vi "Auto Half Ratchet.vi"(9 "ServoDeviceRef":T11, 10 "ServoDeviceRef 2":T11, 11 "RobotDriveDevRef":T1) -> ()   [LabVIEW 2014]
uses:
  <vilib>/Rock Robotics/WPI/PWM/Servo/WPI_ServoDeviceRef.ctl
  <vilib>/Rock Robotics/SystemInterfaces/Typedef/FPGA_TypedefDigitalModule.ctl
  <vilib>/Rock Robotics/SystemInterfaces/DIO/FPGA_DIOPWMChannel.ctl
  <vilib>/Rock Robotics/WPI/PWM/WPI_PWMDeadband.ctl
  <vilib>/Rock Robotics/WPI/RobotDrive/WPI_RobotDriveDevRef.ctl
  <vilib>/Rock Robotics/WPI/MotorControl/WPI_MotorControlDeviceRef.ctl
  <vilib>/Rock Robotics/WPI/MotorControl/WPI_MotorControlType.ctl
  <vilib>/Rock Robotics/WPI/CAN/Jaguar/SubVIs/WPI_CANJaguar_ControlMode.ctl
  <vilib>/Rock Robotics/WPI/CAN/TalonSRX/WPI_CANTalonSRX_APIControlMode.ctl
  <vilib>/Rock Robotics/WPI/PWM/WPI_PWMTransform_ConPane.ctl
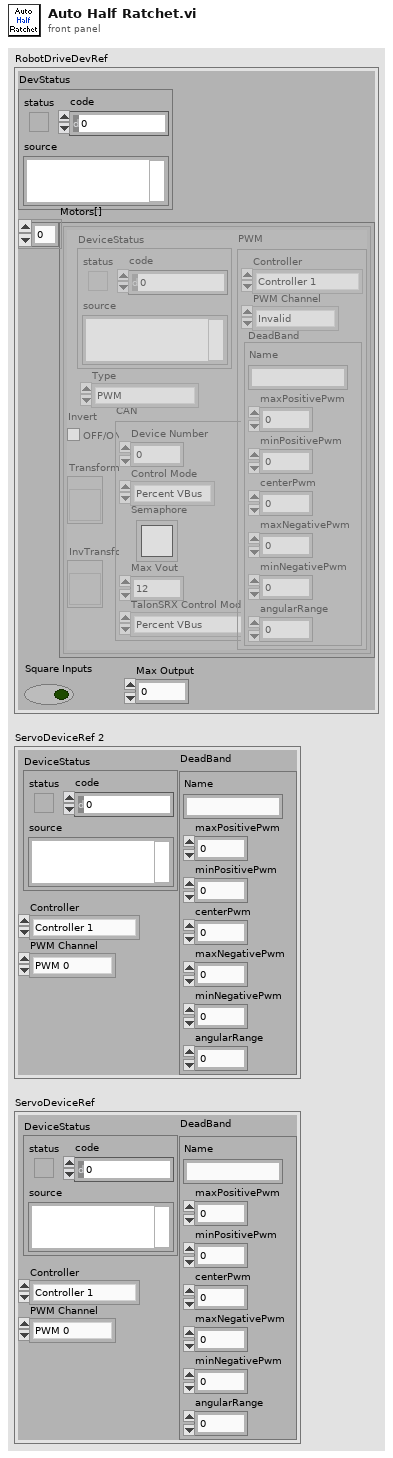
[diagram p1: front panel]
types:
  T1 = typedef "WPI_RobotDriveDevRef.ctl" = cluster{"DevStatus":errorcluster, "Motors[]":T2[], "Square Inputs":bool, "Max Output":dbl}
  T2 = typedef "WPI_MotorControlDeviceRef.ctl" = cluster{"DeviceStatus":errorcluster, "Type":T3, "PWM":cluster{"Controller":T4, "PWM Channel":T5, "DeadBand":T6}, "CAN":cluster{"Device Number":u8, "Control Mode":T7, "Semaphore":T8, "Max Vout":dbl, "TalonSRX Control Mode":T9}, "Invert":bool, "TransformRef":T10, "InvTransformRef":T10}
  T3 = typedef "WPI_MotorControlType.ctl" = enum16{"PWM", "CAN", "CANTalonSRX"}
  T4 = typedef "FPGA_TypedefDigitalModule.ctl" = enum16{"Controller 1"}
  T5 = typedef "FPGA_DIOPWMChannel.ctl" = enum8{"PWM 0", "PWM 1", "PWM 2", "PWM 3", "PWM 4", "PWM 5", "PWM 6", "PWM 7", "PWM 8", "PWM 9", "PWM MXP 0", "PWM MXP 1", "PWM MXP 2", "PWM MXP 3", "PWM MXP 4", "PWM MXP 5", "PWM MXP 6", "PWM MXP 7", "PWM MXP 8", "PWM MXP 9", "Invalid"}
  T6 = typedef "WPI_PWMDeadband.ctl" = cluster{"Name":string, "maxPositivePwm":i32, "minPositivePwm":i32, "centerPwm":i32, "maxNegativePwm":i32, "minNegativePwm":i32, "angularRange":u16}
  T7 = typedef "WPI_CANJaguar_ControlMode.ctl" = enum8{"Percent VBus", "Current", "Speed", "Position", "Voltage"}
  T8 = typedef "Semaphore RefNum" = refnum<k1>
  T9 = typedef "WPI_CANTalonSRX_APIControlMode.ctl" = enum8{"Percent VBus", "Speed", "Position", "Slave", "Unchanged / Invalid"}
  T10 = typedef "WPI_PWMTransform_ConPane.ctl" = refnum<vi>
  T11 = typedef "WPI_ServoDeviceRef.ctl" = cluster{"DeviceStatus":errorcluster, "Controller":T4, "PWM Channel":T5, "DeadBand":T6}
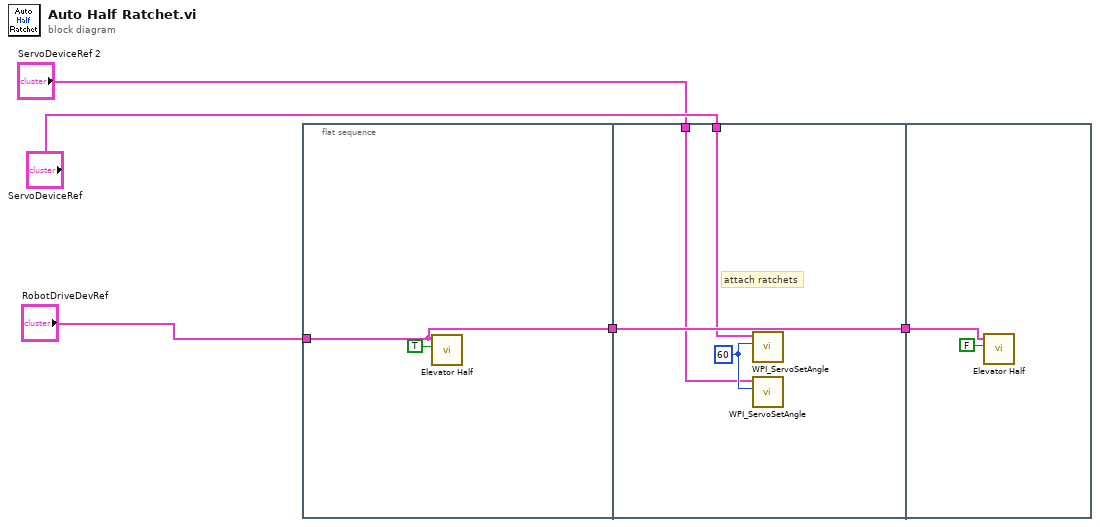
[diagram p0: block diagram]
diagram:
  n1 = flat-sequence {
    tunnel: "RobotDriveDevRef" -> [w6]
    tunnel: [w6] -> w5
    tunnel: [w11] -> w4
    tunnel: w5 -> [w11]
    tunnel: "ServoDeviceRef 2" -> [w9]
    tunnel: "ServoDeviceRef" -> [w8]
    tunnel: w4 -> [w12]
    frame #0 {
      n2 = call "Elevator Half.vi"("Forward?"=TRUE, "RobotDriveDevRef in"=w6) -> ()  [unwired: 10 in]
    }
    frame #1 {
      w10 = 60 ("Angle")
      # "attach ratchets"
      n3 = call <vilib>:"WPI_ServoSetAngle.vi"("Angle"=w10, "ServoDeviceRef"=w8) -> ()  [unwired: 8 in, 2 out]
      n4 = call <vilib>:"WPI_ServoSetAngle.vi"("Angle"=w10, "ServoDeviceRef"=w9) -> ()  [unwired: 8 in, 2 out]
    }
    frame #2 {
      n5 = call "Elevator Half.vi"("Forward?"=FALSE, "RobotDriveDevRef in"=w12) -> ()  [unwired: 10 in]
    }
  }
